vi "ConvertWEBPtoJPG.vi"(8 "error in":errorcluster, 11 "Working Path":path) -> (0 "error out":errorcluster, 3 "Working Path Out":path)   [LabVIEW 2024]
uses:
  <userlib>/_OpenG.lib/file/file.llb/Convert File Extension (Path)__ogtk.vi
  <userlib>/_OpenG.lib/file/file.llb/openg_file.lvlib
panel:
  out "current":string
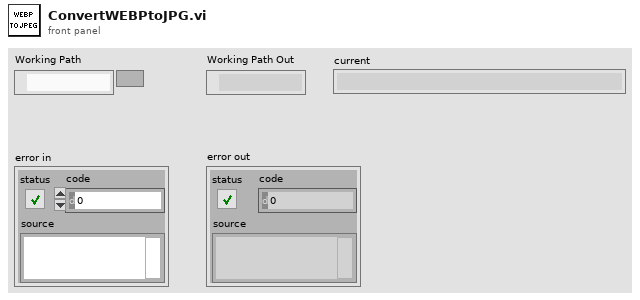
[diagram p1: front panel]
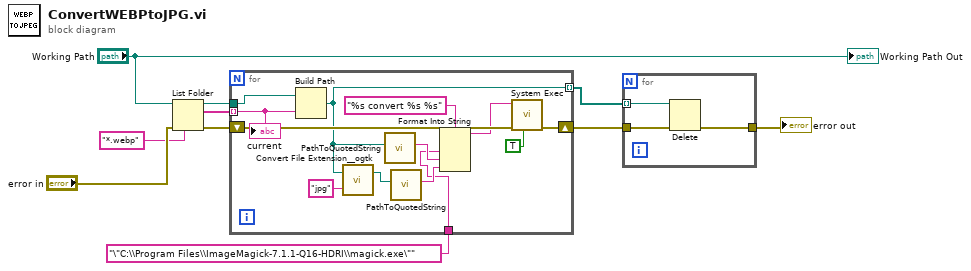
[diagram p0: block diagram]
diagram:
  n1 = List Folder(path="Working Path", pattern="*.webp", error in="error in") -> (path out=w7:path, filenames=w5:string[], error out=w6:errorcluster)  [unwired: 1 in, 1 out]
  n2 = for {
    tunnel: w7 -> [w22]
    shift-right: [w11] -> w3
    shift-left: w6 -> [w19]
    tunnel: w5 -> [w23] mode=indexing
    tunnel: "\"C:\\Program Files\\ImageMagick-7.1.1-Q16-HDRI\\magick.exe\"" -> [w13]
    tunnel: [w12] -> w2 mode=indexing
    n3 = Build Path(base path=w22, name or relative path=w23) -> (appended path=w12:path)
    n4 = call-poly <userlib>:"Convert File Extension__ogtk.vi"("new ending (none)"="jpg", "file name"=w12) -> ("new filename"=w15:path)  [unwired: 1 out]
    n5 = call "PathToQuotedString.vi"("Path"=w12) -> ("String"=w16:string)  [unwired: 10 in]
    n6 = call "PathToQuotedString.vi"("Path"=w15) -> ("String"=w14:string)  [unwired: 10 in]
    n7 = Format Into String(format string="%s convert %s %s", w13, w16, w14) -> (resulting string=w17:string)  [unwired: 2 in, 1 out]
    n8 = call <vilib>:"System Exec.vi"("run minimized? (F)"=TRUE, "error in (no error)"=w19, "command line"=w17) -> ("error out"=w11:errorcluster)  [unwired: 5 in, 3 out]
    "current" <- w23
  }
  n9 = for {
    tunnel: w2 -> [w24] mode=indexing
    tunnel: w3 -> [w26]
    tunnel: [w25] -> w1
    n10 = Delete(path (use dialog)=w24, error in=w26) -> (error out=w25:errorcluster)  [unwired: 3 in, 2 out]
  }
  "error out" <- w1
  "Working Path Out" <- "Working Path"
